vi "Queue Init.vi"(9 "Queue Self":map{string, refnum<data-value>}(c390), 10 "Queue Caller":map{string, refnum<data-value>}(c390)) -> (3 "Base Queue jettl out":refnum<class "Base Queue jettl.lvclass">)   [LabVIEW 2021, in "jettl.lvlib" / "Base Queue jettl.lvlib" / "Base Queue jettl.lvclass"]
uses:
  Base Queue jettl.lvclass
  Msg/Msg/Msg.lvclass
  State/Nominal State/Nominal State.lvclass
  C:/git/jettl/src/jettl/Base Queue jettl/State/State/State.lvclass
  Base Queue jettl.lvclass/Base Queue jettl.ctl
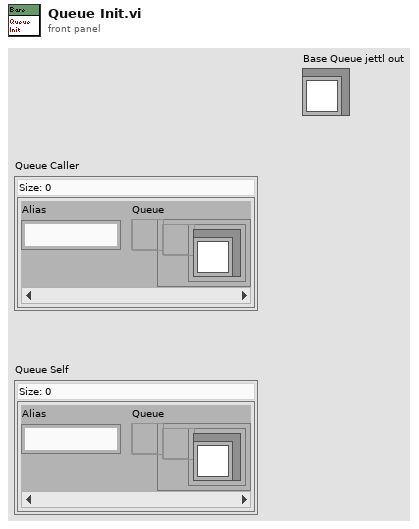
[diagram p1: front panel]
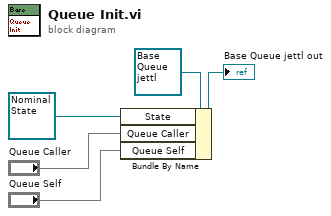
[diagram p0: block diagram]
diagram:
  n1 = Bundle By Name(cluster=refnum<class "Base Queue jettl.lvclass"> refnum ("Self Actor in"), "State"=refnum<class "Nominal State.lvclass"> refnum ("jettl.lvlib:Nominal Queue State.lvclass"), "Queue Caller"="Queue Caller", "Queue Self"="Queue Self") -> (→"Base Queue jettl out":refnum<class "Base Queue jettl.lvclass">)
